vi "InitialPortsGuiUpdater.vi"(0 "Ports counter":i32, 1 "port max size":i32, 2 "MCListbox Refnum":refnum<vi>) -> ()   [LabVIEW 2009]
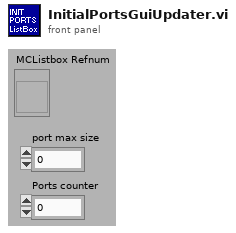
[diagram p1: front panel]
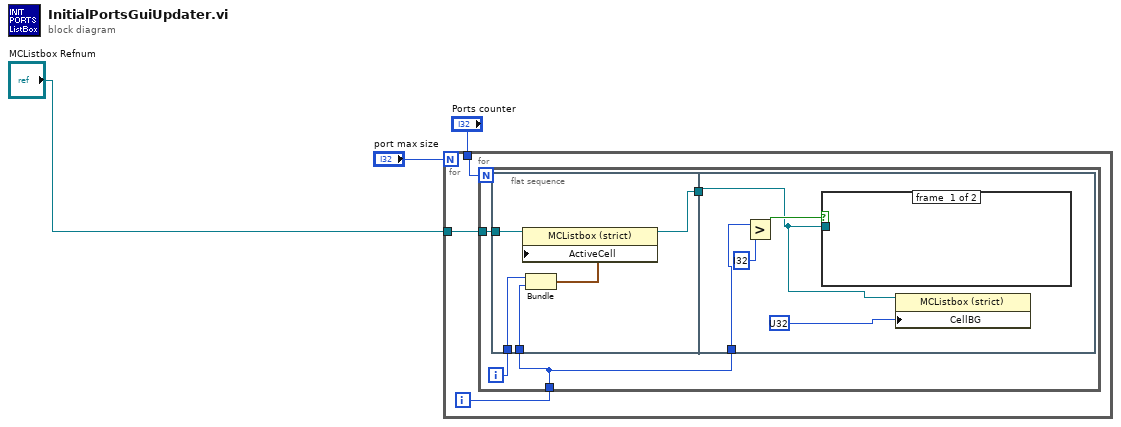
[diagram p0: block diagram]
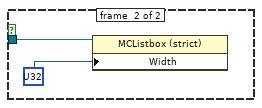
[diagram p2: hidden frame]
diagram:
  n1 = for {
    N: "port max size" -> [_]
    tunnel: "Ports counter" -> [w6]
    tunnel: "MCListbox Refnum" -> [w4]
    i -> [w5]
    n2 = for {
      N: w6 -> [_]
      tunnel: w5 -> [w9]
      tunnel: w4 -> [w8]
      i -> [w10]
      n3 = flat-sequence {
        tunnel: w10 -> [w14]
        tunnel: w9 -> [w13]
        tunnel: w8 -> [w12]
        tunnel: [w11] -> w7
        tunnel: w9 -> [w18]
        tunnel: w7 -> [w16]
        frame #0 {
          n4 = Bundle(w14, w13) -> (w15:cluster{i32, i32})  [unwired: 1 in]
          n5 = property on="Property Node" class="MCListbox (strict)"(reference=w12, "ActiveCell"=w15) -> (reference out=w11:refnum<vi>)  [unwired: 1 in, 1 out]
        }
        frame #1 {
          n6 = Greater?(x=w18, y=i32 ?) -> (0:w19:bool)
          n7 = case shown="True" w19 {
            tunnel: w16 -> [_ w21]
            frame #0 {
            }
            frame #1 {
              n8 = property on="Property Node" class="MCListbox (strict)"(reference=w21, "Width"=u32 ? ("Cell Size:Width")) -> ()  [unwired: 1 in, 2 out]
            }
          }
          n9 = property on="Property Node" class="MCListbox (strict)"(reference=w16, "CellBG"=u32 ? ("Cell Background Color")) -> ()  [unwired: 1 in, 2 out]
        }
      }
    }
  }
